vi "sub vi - QPD channels 2.vi"(1 "Include Position?":bool) -> (8 "QPD Channels":tag="Dev3/ai21,Dev3/ai22,Dev3/ai23,Dev3/ai19")   [LabVIEW 2010]
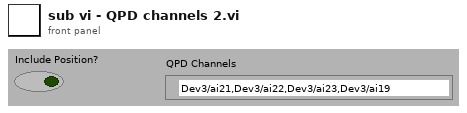
[diagram p1: front panel]
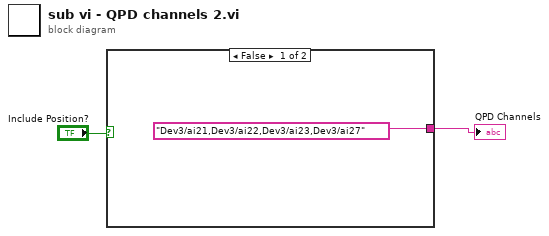
[diagram p0: block diagram]
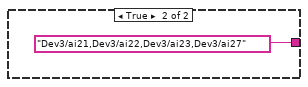
[diagram p2: hidden frame]
diagram:
  n1 = case shown="False" "Include Position?" {
    tunnel: [tag "Dev3/ai21,Dev3/ai22,Dev3/ai23,Dev3/ai27" ("physical channels") tag "Dev3/ai21,Dev3/ai22,Dev3/ai23,Dev3/ai27" ("physical channels")] -> w1
    frame False {
    }
    frame True {
    }
  }
  "QPD Channels" <- w1
